vi "close.vi"(8 "error in (no error)":errorcluster, 11 "Xcite in":refnum<class "Xcite.lvclass">) -> (0 "error out":errorcluster)   [LabVIEW 2019, in "Xcite.lvclass"]
doc: "Turns off any output and closes communications with the XCite device."
uses:
  Xcite.lvclass
  Xcite.lvclass/Xcite.ctl
  etc.xcite/XCite.lvlib
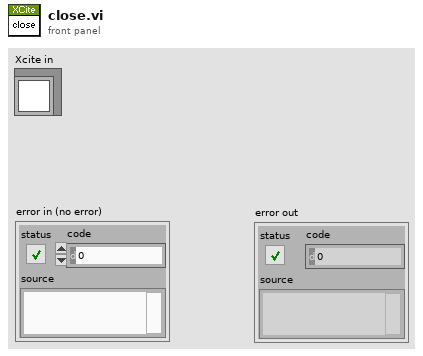
[diagram p1: front panel]
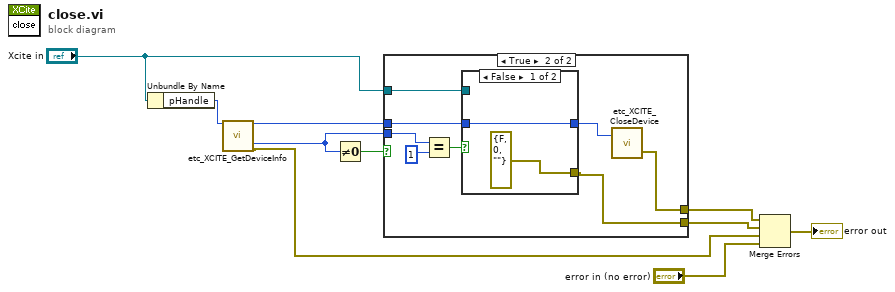
[diagram p0: block diagram]
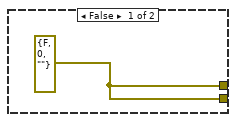
[diagram p2: hidden frame]
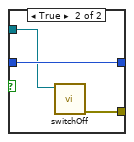
[diagram p3: hidden frame]
diagram:
  n1 = Unbundle By Name("Xcite in") -> ("pHandle"=w9:u64)
  n2 = call "etc_XCITE_GetDeviceInfo.vi"("h"=w9) -> ("h out"=w8:u64, "open_count"=w1:u32, "error out"=w5:errorcluster)  [unwired: 13 in, 3 out]
  n3 = Not Equal To 0?(x=w1) -> (x != 0?=w7:bool)
  n4 = case shown="True" w7 {
    tunnel: w8 -> [_ w15]
    tunnel: [w11 w19] -> w2
    tunnel: w1 -> [_ w16]
    tunnel: "Xcite in" -> [_ w13]
    tunnel: [w11 w12] -> w3
    frame False {
      w11 = errorcluster {"status"=FALSE, "code"=0, "source"=""} ("error out")
    }
    frame True {
      n5 = Equal?(x=w16, y=u32 1) -> (x = y?=w17:bool)
      n6 = case shown="False" w17 {
        tunnel: w15 -> [w21 w24]
        tunnel: [w21 w24] -> w14
        tunnel: [errorcluster {"status"=FALSE, "code"=0, "source"=""} ("error _out") w23] -> w12
        tunnel: w13 -> [_ w22]
        frame False {
        }
        frame True {
          n7 = call "switchOff.vi"("Xcite in"=w22) -> ("error out"=w23:errorcluster)  [unwired: 9 in, 1 out]
        }
      }
      n8 = call "etc_XCITE_CloseDevice.vi"("h"=w14) -> ("error out"=w19:errorcluster)  [unwired: 2 in]
    }
  }
  n9 = Merge Errors(w2, w3, w5, "error in (no error)") -> (→"error out":errorcluster)
